vi "Apply.vi"(8 "error in":errorcluster, 11 "Thermometer DAQmx RTD Cont CFG in":refnum<class "Thermometer DAQmx RTD Cont CFG.lvclass">) -> (0 "error out":errorcluster, 3 "Thermometer DAQmx RTD Cont CFG out":refnum<class "Thermometer DAQmx RTD Cont CFG.lvclass">)   [LabVIEW 2023, in "Thermometer DAQmx RTD Cont CFG.lvclass"]
uses:
  Thermometer DAQmx RTD Cont CFG.lvclass
  Thermometer DAQmx RTD Cont CFG.lvclass/Thermometer DAQmx RTD Cont CFG.ctl
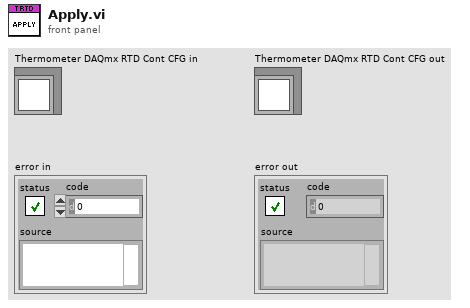
[diagram p1: front panel]
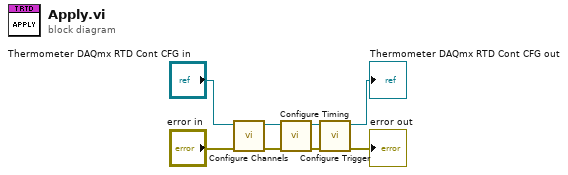
[diagram p0: block diagram]
diagram:
  n1 = call-dynamic "Configure Channels.vi"("error in"="error in", "Thermometer DAQmx RTD Cont CFG in"="Thermometer DAQmx RTD Cont CFG in") -> ("error out"=w7:errorcluster, "Thermometer DAQmx RTD Cont CFG out"=w6:refnum<class "Thermometer DAQmx RTD Cont CFG.lvclass">)  [unwired: 8 in]
  n2 = call-dynamic "Configure Timing.vi"("error in"=w7, "DAQmx Base CFG in"=w6) -> ("error out"=w5:errorcluster, "DAQmx Base CFG out"=w3:refnum<class "Thermometer DAQmx RTD Cont CFG.lvclass">)  [unwired: 8 in]
  n3 = call-dynamic "Configure Trigger.vi"("error in"=w5, "DAQmx Base CFG in"=w3) -> ("error out"=→"error out":errorcluster, "DAQmx Base CFG out"=→"Thermometer DAQmx RTD Cont CFG out":refnum<class "Thermometer DAQmx RTD Cont CFG.lvclass">)  [unwired: 8 in]
